vi "NormalizedPositionAverage.vi"(11 "f":dbl) -> (3 "mean":dbl)   [LabVIEW 2015]
uses:
  <vilib>/Analysis/baseanly.llb/Mean (DBL).vi
  <vilib>/Analysis/NI_AALBase.lvlib
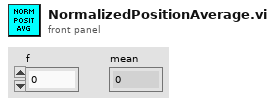
[diagram p1: front panel]
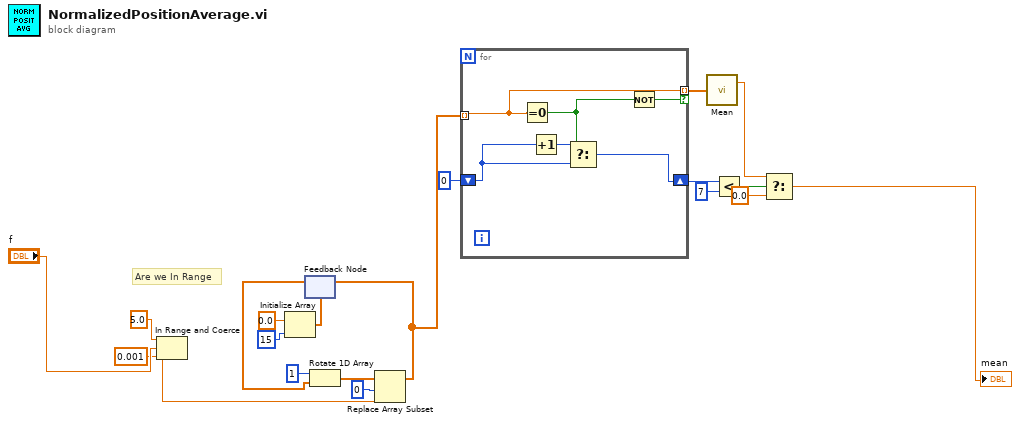
[diagram p0: block diagram]
diagram:
  # "Are we In Range"
  n1 = In Range and Coerce(upper limit=5.0, x="f", lower limit=0.001) -> (coerced(x)=w10:dbl)  [unwired: 1 out]
  n2 = Initialize Array(0.0 ("element"), 15 ("dimension size")) -> (w11:dbl[])
  n3 = feedback #1(w11) -> (w12:dbl[])
  n4 = Rotate 1D Array(1:w12, 2:1 ("n")) -> (0:w14:dbl[])
  n5 = Replace Array Subset(array=w14, new element=w10, index=0) -> (w1:dbl[])
  n6 = feedback-in #1(w1) -> ()
  n7 = for {
    tunnel: w1 -> [w23] mode=indexing
    shift-right: [w24] -> w8
    shift-left: 0 -> [w26]
    tunnel: [w23] -> w4 mode=indexing if=w21
    n8 = Equal To 0?(x=w23) -> (x = 0?=w22:bool)
    n9 = Increment(x=w26) -> (x+1=w25:i32)
    n10 = Select(t=w25, s=w22, f=w26) -> (s? t:f=w24:i32)
    n11 = Not(x=w22) -> (.not. x?=w21:bool)
  }
  n12 = call-poly <vilib>:"Mean.vi"("X"=w4) -> ("mean"=w3:dbl)  [unwired: 1 out]
  n13 = Less?(x=w8, y=7) -> (x < y?=w6:bool)
  n14 = Select(t=w3, s=w6, f=0.0) -> (s? t:f=→"mean":dbl)
